vi "Can Teardown Init.vi"(8 "Error in":errorcluster, 10 "Actor in":refnum<class "Actor.lvclass">) -> (1 "Teardown Init":bool, 2 "Actor out":refnum<class "Actor.lvclass">)   [LabVIEW 2020, in "jettl.lvlib" / "Actor.lvlib"]
uses:
  Actor.lvlib
  Actor/Actor.lvclass
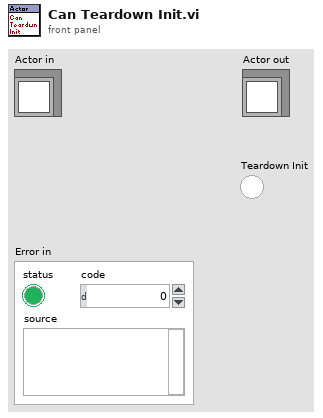
[diagram p1: front panel]
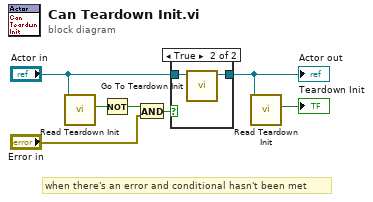
[diagram p0: block diagram]
diagram:
  # "when there's an error and conditional hasn't been met"
  n1 = call-dynamic "Read Teardown Init.vi"("Actor in"="Actor in") -> ("Teardown Init"=w7:bool)  [unwired: 10 in]
  n2 = Not(x=w7) -> (.not. x?=w3:bool)
  n3 = And(x=w3, y="Error in") -> (x .and. y?=w2:bool)
  n4 = case shown="True" w2 {
    tunnel: [w8 w9] -> w5
    tunnel: "Actor in" -> [w8 w10]
    frame False {
    }
    frame True {
      n5 = call-dynamic "Go To Teardown Init.vi"("Actor in"=w10) -> ("Actor out"=w9:refnum<class "Actor.lvclass">)  [unwired: 10 in]
    }
  }
  "Actor out" <- w5
  n6 = call-dynamic "Read Teardown Init.vi"("Actor in"=w5) -> ("Teardown Init"=→"Teardown Init":bool)  [unwired: 10 in]
